vi "Get as LabVIEW Text.vi"(8 "error in (no error)":errorcluster, 10 "Name Array":string[](array[string]), 11 "JSON Value In":refnum<class "JSON Value.lvclass">) -> (0 "error out":errorcluster, 1 "Was in quotes":bool, 2 "LabVIEW Text":string, 3 "JSON Value Out":refnum<class "JSON Value.lvclass">)   [LabVIEW 2020, in "Library Commun.lvlib" / "JSON Value.lvclass"]
uses:
  JSON Value.lvclass
panel:
  # "Value formated as LabVIEW text:\n-- no quotes on JSON strings\n-- LabVIEW text encoding <ToDo>\n-- no escaped characters <ToDo>"
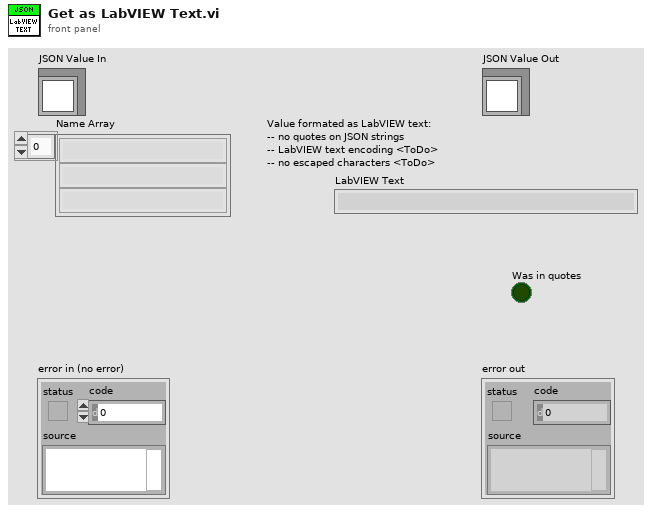
[diagram p1: front panel]
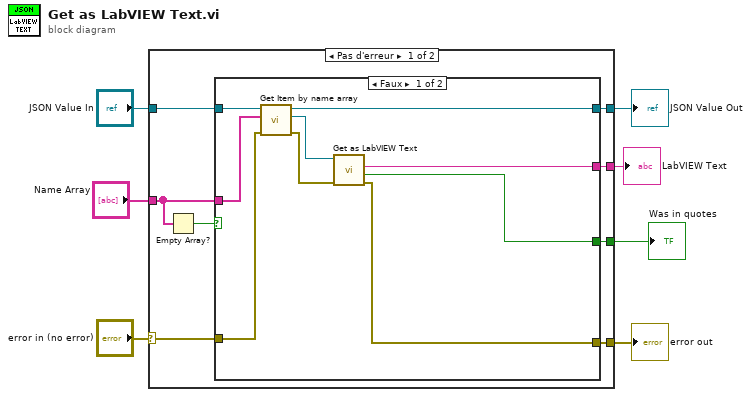
[diagram p0: block diagram]
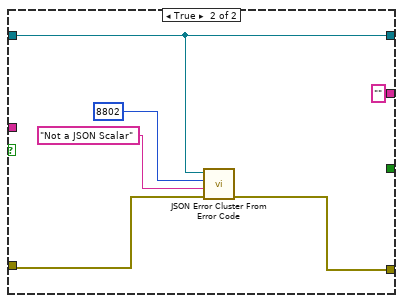
[diagram p2: hidden frame]
diagram:
  n1 = case shown="Pas d'erreur" "error in (no error)" {
    selector: "error in (no error)" -> [w14 w32]
    tunnel: [w13 w32] -> w6
    tunnel: [w10 w31] -> w4
    tunnel: "JSON Value In" -> [w12 w31]
    tunnel: [w15 _] -> w3
    tunnel: "Name Array" -> [w9 _]
    tunnel: [w8 _] -> w1
    frame No Error {
      n2 = Empty Array?(array=w9) -> (empty?=w11:bool)
      n3 = case shown="Faux" w11 {
        tunnel: [w20 ""] -> w15
        tunnel: w14 -> [w17 w27]
        tunnel: [w18 w26] -> w13
        tunnel: w12 -> [w24 w25]
        tunnel: [w22 w25] -> w10
        tunnel: w9 -> [w23 _]
        tunnel: [w16 _] -> w8
        frame False {
          n4 = call "Get Item by name array.vi"("error in (no error)"=w17, "Name Array"=w23, "JSON Value In"=w24) -> ("error out"=w19:errorcluster, "Value"=w21:refnum<class "JSON Value.lvclass">, "JSON Value Out"=w22:refnum<class "JSON Value.lvclass">)  [unwired: 5 in, 1 out]
          n5 = call-dynamic "Get as LabVIEW Text.vi"("error in (no error)"=w19, "JSON Value In"=w21) -> ("error out"=w18:errorcluster, "Was in quotes"=w16:bool, "LabVIEW Text"=w20:string)  [unwired: 6 in, 1 out]
        }
        frame True {
          n6 = call "JSON Error Cluster From Error Code.vi"("error in (no error)"=w27, "Error message"="Not a JSON Scalar", "JSON error code"=8802, "JSON Value in"=w25) -> ("error out"=w26:errorcluster)  [unwired: 6 in, 1 out]
        }
      }
    }
    frame Error {
    }
  }
  "error out" <- w6
  "JSON Value Out" <- w4
  "LabVIEW Text" <- w3
  "Was in quotes" <- w1
